vi "DUC (One Channel).vi"(0 "data":u32, 1 "reset":bool, 5 "enable":bool, 9 "input valid":bool, 11 "duc parameters":T1={"frequency shift"=0.0, "impairments"={"inline gain I"=0.9999923706054688, "inline gain Q"=0.9999923706054688, "cross gain I"=0.0, "cross gain Q"=0.0, "pre-gain offset I"=0.0, "pre-gain offset Q"=0.0, "post-gain offset I"=0.0, "post-gain offset Q"=0.0}, "phase"=0.0, "input sample rate"=0.0, "gain"={"gain I"=1.0, "gain Q"=1.0}, "delay"=0.0} {"frequency shift" format="%#.48g"}) -> (4 "I data out":i16, 6 "Q data out":i16, 10 "output valid":bool, 13 "dsp reset done":bool, 14 "ready for input":bool, 15 "number of overflows":u64)   [LabVIEW 2021]
doc: "Digital upconverter (DUC). Implemented with FPGA-based DSP.\n\n<B>Input Parameters</B>\n\n<B>data in</B> is the I and Q data to be upconverted along with overflow information.\n\n<B>enable</B> specifies which streams are enabled.\n\n<B>input valid</B> specifies when 'data in' is valid.\n\n<B>duc parameters</B> are the upconversion parameters utilized by the DSP chain.\n\n<B>reset</B> the DSP upconversion signal chain.\n\n<B>Output Parameters</B>\n\n<B>dsp reset done</B> indicates that the DSP upconversion signal chain completed reset.\n\n<B>ready for input</B> is a flow control signal that indicates whether the DUC is ready to accept new data.\n\n<B>I data out</B> is the in phase component of upconverted data to be transmitted.\n\n<B>Q data out</B> is the quadrature phase component of upconverted data to be transmitted.\n\n<B>output valid</B> specifies when 'data out' is valid.\n\n<B>number of overflows</B> is the number of times the DSP chain overflowed on fixed point conversion of 'data in'."
uses:
  DUC Parameters.ctl
  <instrlib>/_niInstr/DSP/v1/Shared/Public/IQ Impairments.ctl
  <instrlib>/_niInstr/DSP/v1/Shared/Public/IQ Gain.ctl
  <instrlib>/_niInstr/DSP/v1/Shared/Public/IQ Data.ctl
  <instrlib>/_niInstr/DSP/v1/FPGA/Public/Sub VIs/Data Conversion/U32 to IQ - 1 spc - S18.1.vi
  <instrlib>/_niInstr/Basic Elements/v1/FPGA/Private/Count Up U64.vi
  <instrlib>/_niInstr/DSP/v1/FPGA/Public/Sub VIs/Digital Gain/Digital Gain - 1 spc.vi
  <instrlib>/_niInstr/DSP/v1/FPGA/Public/Sub VIs/Fractional Interpolator/Fractional Interpolator - 1 spc - 2x oc.vi
  <instrlib>/_niInstr/DSP/v1/FPGA/Public/Sub VIs/Frequency Shift/Frequency Shift - 1 spc.vi
  <instrlib>/_niInstr/DSP/v1/FPGA/Public/Sub VIs/IQ Impairments/IQ Impairments - 1 spc.vi
  <instrlib>/_niInstr/DSP/v1/FPGA/Public/Sub VIs/Data Conversion/IQ to I16 - 1 spc - S18.1.vi
  <instrlib>/_niInstr/Basic Elements/v1/FPGA/niInstr Basic Elements v1 FPGA.lvlib
  <instrlib>/_niInstr/DSP/v1/FPGA/niInstr DSP v1 FPGA.lvlib
  <instrlib>/_niInstr/DSP/v1/Shared/niInstr DSP v1 Shared.lvlib
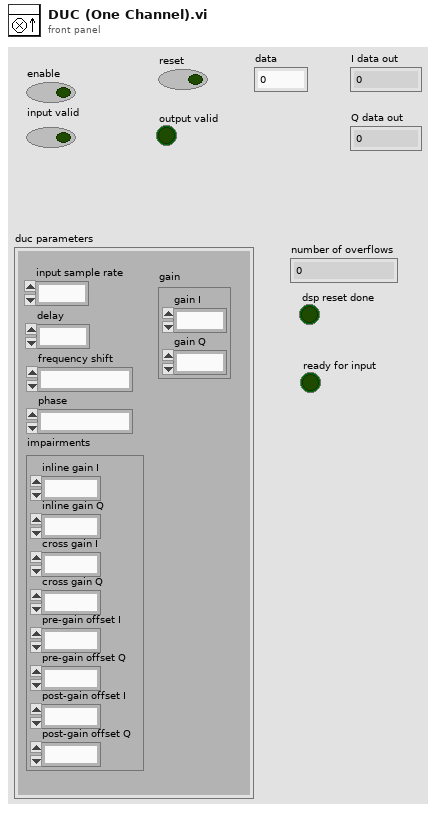
[diagram p1: front panel]
types:
  T1 = typedef "DUC Parameters.ctl" = cluster{"frequency shift":fxp<+/-,48,0>, "impairments":T2, "phase":fxp<+/-,21,0>, "input sample rate":fxp<+,48,1>, "gain":T3, "delay":fxp<+/-,18,0>}
  T2 = typedef "niInstr DSP v1 Shared.lvlib/IQ Impairments.ctl" = cluster{"inline gain I":fxp<+/-,18,1>, "inline gain Q":fxp<+/-,18,1>, "cross gain I":fxp<+/-,18,1>, "cross gain Q":fxp<+/-,18,1>, "pre-gain offset I":fxp<+/-,18,1>, "pre-gain offset Q":fxp<+/-,18,1>, "post-gain offset I":fxp<+/-,18,1>, "post-gain offset Q":fxp<+/-,18,1>}
  T3 = typedef "niInstr DSP v1 Shared.lvlib/IQ Gain.ctl" = cluster{"gain I":fxp<+/-,24,3>, "gain Q":fxp<+/-,24,3>}
  T4 = typedef "niInstr DSP v1 Shared.lvlib/IQ Data.ctl" = cluster{"I":fxp<+/-,18,1>, "Q":fxp<+/-,18,1>, "overflow":bool}
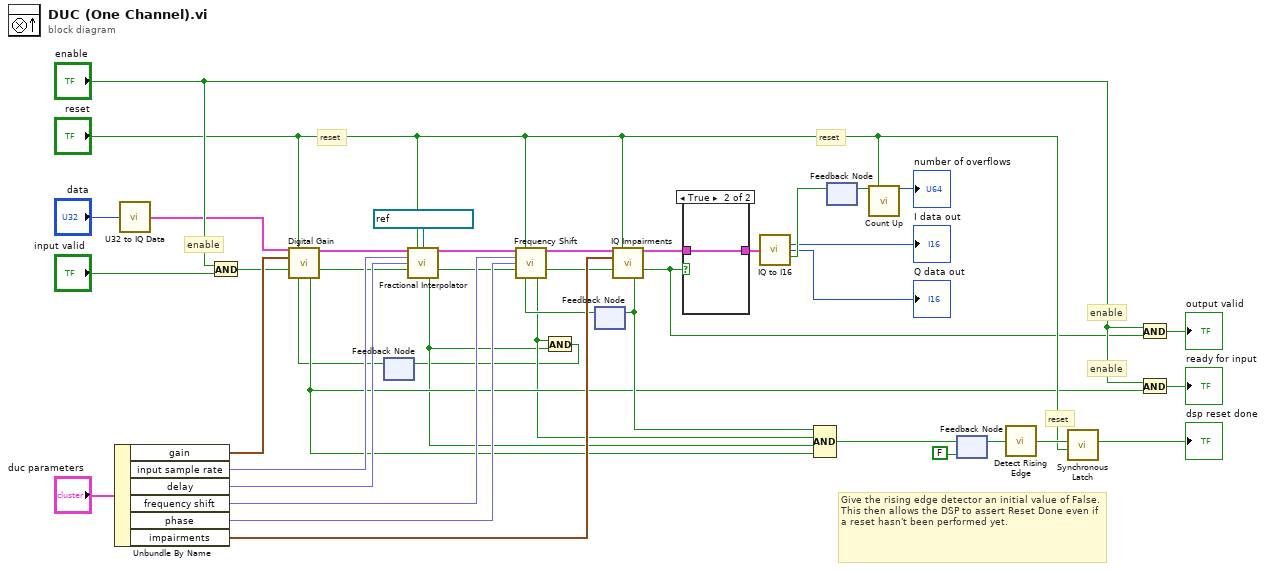
[diagram p0: block diagram]
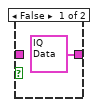
[diagram p2: hidden frame]
diagram:
  # "Give the rising edge detector an initial value of False.  This then allows the DSP to assert Reset Done even if a reset hasn't been performed yet."
  # "enable"
  # "reset"
  # "reset"
  # "reset"
  # "enable"
  # "enable"
  n1 = Unbundle By Name("duc parameters") -> ("gain"=w34:T3, "input sample rate"=w28:fxp<+,48,1>, "delay"=w27:fxp<+/-,18,0>, "frequency shift"=w26:fxp<+/-,48,0>, "phase"=w25:fxp<+/-,21,0>, "impairments"=w24:T2)
  n2 = call-poly <instrlib>:"U32 to IQ Data.vi"("U32 data"="data") -> ("IQ data"=w1:T4)  [unwired: 14 in]
  n3 = And(x="enable", y="input valid") -> (x .and. y?=w23:bool)
  n4 = feedback #1() -> (w2:bool)  [unwired: 1 in]
  n5 = call-poly <instrlib>:"Digital Gain.vi"("data in"=w1, "reset"="reset", "gain"=w34, "input valid"=w23, "ready for output (T)"=w2) -> ("data out"=w15:T4, "output valid"=w14:bool, "ready for input"=w7:bool)  [unwired: 7 in, 1 out]
  n6 = call-poly <instrlib>:"Fractional Interpolator.vi"("data in"=w15, "reset"="reset", "clock x 2"=refnum<k21> "Data Clock x2" ("oversample clock"), "input sample rate"=w28, "delay"=w27, "input valid"=w14) -> ("data out"=w19:T4, "output valid"=w18:bool, "ready for input"=w4:bool)  [unwired: 6 in, 1 out]
  n7 = feedback #2() -> (w12:bool)  [unwired: 1 in]
  n8 = call-poly <instrlib>:"Frequency Shift.vi"("data in"=w19, "reset"="reset", "frequency shift"=w26, "phase"=w25, "input valid"=w18, "ready for output (T)"=w12) -> ("data out"=w17:T4, "output valid"=w16:bool, "ready for input"=w5:bool)  [unwired: 6 in, 1 out]
  n9 = And(x=w5, y=w4) -> (x .and. y?=w3:bool)
  n10 = feedback-in #1(w3) -> ()
  n11 = call-poly <instrlib>:"IQ Impairments.vi"("data in"=w17, "reset"="reset", "impairments"=w24, "input valid"=w16) -> ("data out"=w21:T4, "output valid"=w22:bool, "ready for input"=w8:bool)  [unwired: 8 in, 1 out]
  n12 = feedback-in #2(w8) -> ()
  n13 = case shown="True" w22 {
    tunnel: w21 -> [_ w44]
    tunnel: [T4 {"I"=0.0, "Q"=0.0, "overflow"=FALSE} ("data out") w44] -> w20
    frame False {
    }
    frame True {
    }
  }
  n14 = call-poly <instrlib>:"IQ to I16.vi"("IQ"=w20) -> ("I"=→"I data out":i16, "Q"=→"Q data out":i16, "overflow"=w31:bool)  [unwired: 12 in]
  n15 = Compound Arithmetic op=AND(w8, w5, w4, w7) -> (w6:bool)
  n16 = feedback #3() -> (w38:bool)  [unwired: 1 in]
  n17 = feedback-in #3(w31) -> ()
  n18 = call-poly <instrlib>:"Count Up.vi"("increment"=w38, "reset"="reset") -> ("count out"=→"number of overflows":u64)  [unwired: 13 in]
  n19 = feedback-in #4(w6) -> ()
  n20 = feedback #4(FALSE ("ready for input")) -> (w10:bool)
  n21 = call <instrlib>:"Detect Rising Edge.vi"("signal"=w10) -> ("edge detected"=w41:bool)  [unwired: 14 in]
  n22 = call <instrlib>:"Synchronous Latch.vi"("clear"="reset", "set"=w41) -> ("out"=→"dsp reset done":bool)  [unwired: 9 in]
  n23 = And(x="enable", y=w22) -> (x .and. y?=→"output valid":bool)
  n24 = And(x="enable", y=w7) -> (x .and. y?=→"ready for input":bool)
